vi "Memory.Array.Numeric.New.vi"(8 "error in (no error)":errorcluster, 11 "Numeric Array in":refnum<class "Memory.Array.Numeric.lvclass">) -> (0 "error out":errorcluster, 3 "Numeric Array out":refnum<class "Memory.Array.Numeric.lvclass">)   [LabVIEW 2016, in "Memory Manager.lvlib" / "Memory.Array.Numeric.lvclass"]
uses:
  Memory.Array.Numeric.lvclass
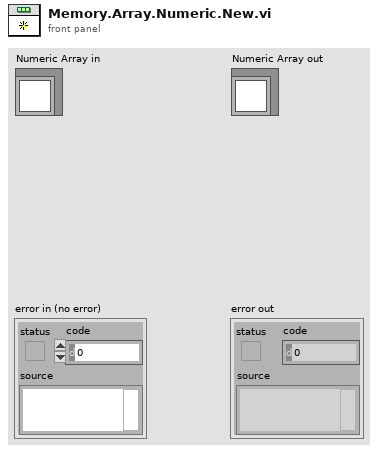
[diagram p1: front panel]
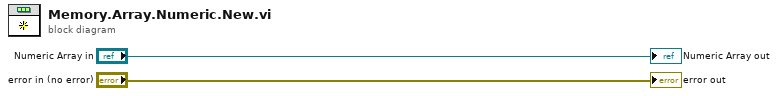
[diagram p0: block diagram]
diagram:
  "error out" <- "error in (no error)"
  "Numeric Array out" <- "Numeric Array in"
